vi "Speed PI Control.vi"() -> ()   [LabVIEW 2015]
panel:
  in  "I-Gain":dbl(slide)=1.0 scale=0.0..2.0
  in  "P-Gain":dbl(slide)=1.0 scale=0.0..2.0
  in  "Setpoint Speed (rps)":dbl(slide) scale=-8.3..8.3
  out "Speed (rps)":dynamicdata(graph)
  in  "stop (F)":bool
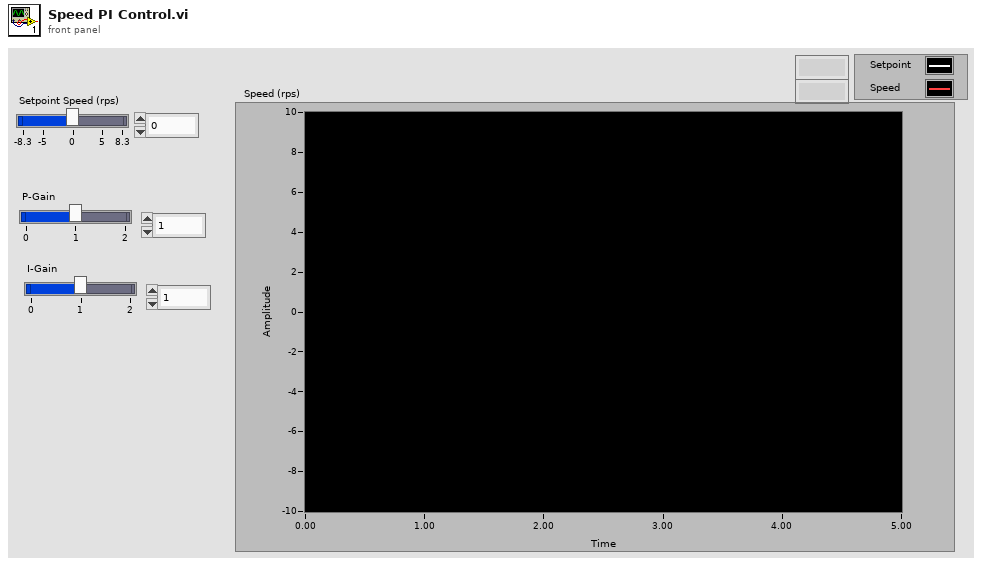
[diagram p1: front panel]
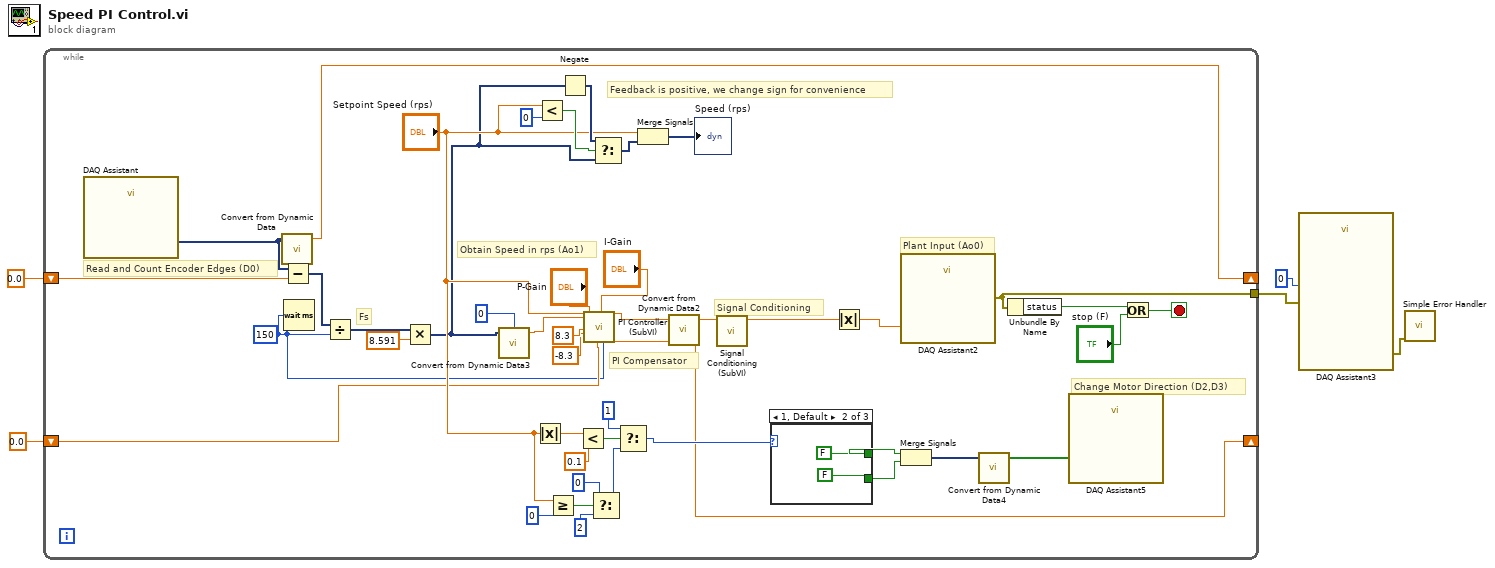
[diagram p0: block diagram]
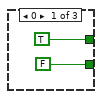
[diagram p2: hidden frame]
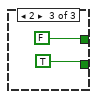
[diagram p3: hidden frame]
diagram:
  n1 = while {
    shift-right: [w49] -> _
    shift-left: 0.0 -> [w48]
    tunnel: [w44] -> w4
    shift-right: [w8] -> _
    shift-left: 0.0 -> [w9]
    stop <- w43 stop-if-true
    w7 = 150
    # "Feedback is positive, we change sign for convenience"
    # "Change Motor Direction (D2,D3)"
    # "Signal Conditioning"
    # "PI Compensator"
    # "Fs"
    # "Obtain Speed in rps (Ao1)"
    # "Read and Count Encoder Edges (D0)"
    # "Plant Input (Ao0)"
    n2 = call "DAQ Assistant"() -> ("data"=w40:dynamicdata)  [unwired: 16 in, 3 out]
    n3 = call "Convert from Dynamic Data"("Dynamic Data Type"=w40) -> ("Scalar"=w49:dbl)  [unwired: 3 in]
    n4 = Subtract(x=w40, y=w48) -> (x-y=w47:dynamicdata)
    n5 = Wait (ms)(milliseconds to wait=w7) -> ()  [unwired: 1 out]
    n6 = Divide(x=w47, y=w7) -> (x/y=w46:dynamicdata)
    n7 = Multiply(x=w46, y=8.591) -> (x*y=w6:dynamicdata)
    n8 = call "Convert from Dynamic Data3"("Dynamic Data Type"=w6, "Channel"=0) -> ("Scalar"=w15:dbl)  [unwired: 2 in]
    n9 = Absolute Value(x="Setpoint Speed (rps)") -> (abs(x)=w30:dbl)
    n10 = Less?(x="Setpoint Speed (rps)", y=0) -> (x < y?=w18:bool)
    n11 = Greater Or Equal?(x="Setpoint Speed (rps)", y=0) -> (x >= y?=w33:bool)
    n12 = Negate(x=w6) -> (-x=w17:dynamicdata)
    n13 = Less?(x=w30, y=0.1) -> (x < y?=w28:bool)
    n14 = call "PI Controller (SubVI).vi"("sp"="Setpoint Speed (rps)", "pv"=w15, "maxim"=8.3, "minim"=-8.3, "p"="P-Gain", "errsum"=w9, "i"="I-Gain", "h"=w7) -> ("output variable"=w12:dbl, "errsum"=w8:dbl)  [unwired: 18 in]
    n15 = Select(t=0, s=w33, f=2) -> (s? t:f=w26:i32)
    n16 = Select(t=w17, s=w18, f=w6) -> (s? t:f=w19:dynamicdata)
    n17 = Select(t=1, s=w28, f=w26) -> (s? t:f=w23:i32)
    n18 = Merge Signals("Setpoint Speed (rps)", w19) -> (→"Speed (rps)":dynamicdata)
    n19 = call "Convert from Dynamic Data2"("Dynamic Data Type"=w12) -> ("Scalar"=w25:dbl)  [unwired: 3 in]
    n20 = call "Signal Conditioning (SubVI).vi"("Input"=w25) -> ("Output"=w22:dbl)  [unwired: 10 in]
    n21 = case shown="1, Default" w23 {
      tunnel: [TRUE FALSE FALSE] -> w36
      tunnel: [FALSE FALSE TRUE] -> w35
      frame 0 {
      }
      frame 1, Default {
      }
      frame 2 {
      }
    }
    n22 = Absolute Value(x=w22) -> (abs(x)=w24:dbl)
    n23 = call "DAQ Assistant2"("data"=w24) -> ("error out"=w44:errorcluster)  [unwired: 17 in, 1 out]
    n24 = Merge Signals(w36, w35) -> (w38:dynamicdata)
    n25 = call "Convert from Dynamic Data4"("Dynamic Data Type"=w38) -> ("Array"=w37:bool[])  [unwired: 3 in]
    n26 = Unbundle By Name(w44) -> ("status"=w41:bool)
    n27 = call "DAQ Assistant5"("data"=w37) -> ()  [unwired: 17 in, 2 out]
    n28 = Or(x=w41, y="stop (F)") -> (x .or. y?=w43:bool)
  }
  n29 = call "DAQ Assistant3"("data"=0, "error in"=w4) -> ("error out"=w2:errorcluster)  [unwired: 16 in, 1 out]
  n30 = call <vilib>:"Simple Error Handler.vi"("error in (no error)"=w2) -> ()  [unwired: 4 in, 5 out]
